vi "ImagenBinarizada.vi"(11 "Refnum in":T1) -> (3 "Refnum out":T1(plugin-control))   [LabVIEW 2021]
uses:
  <vilib>/vision/Image Controls.llb/IMAQ Image.ctl
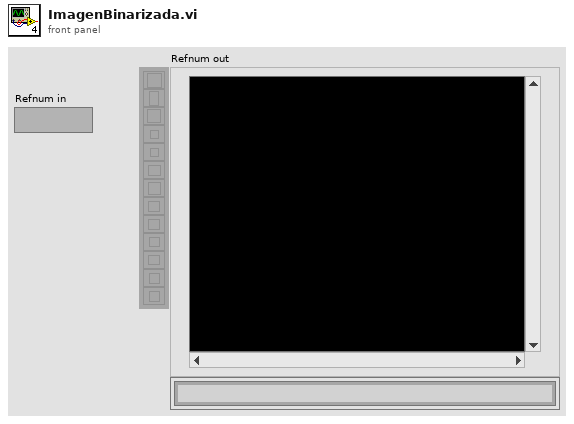
[diagram p1: front panel]
types:
  T1 = typedef "IMAQ Image.ctl" = refnum<image>
  T2 = typedef "Image Type" = u32
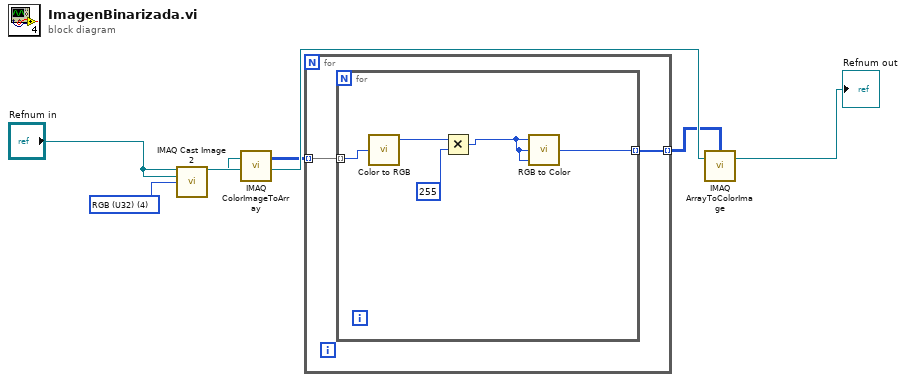
[diagram p0: block diagram]
diagram:
  w1 = T2 4 items=["Grayscale (U8)", "Grayscale (I16)", "Grayscale (SGL)", "Complex (CSG)", "RGB (U32)", "HSL (U32)", "RGB (U64)", "Grayscale (U16)"] ("Image Type")
  n1 = call "IMAQ Cast Image 2"("Image Src"="Refnum in", "Image Dst"="Refnum in", "Image Type"=w1) -> ("Image Dst Out"=w2:T1)  [unwired: 11 in, 1 out]
  n2 = call "IMAQ ColorImageToArray"("Image"=w2) -> ("Image Pixels (U32)"=w3:u32[][])  [unwired: 3 in, 2 out]
  n3 = for {
    tunnel: w3 -> [w8] mode=indexing
    tunnel: [w7] -> w4 mode=indexing
    n4 = for {
      tunnel: w8 -> [w13] mode=indexing
      tunnel: [w9] -> w7 mode=indexing
      n5 = call <vilib>:"Color to RGB.vi"("Color"=w13) -> ("Resolved Color"=w12:u32)  [unwired: 3 out]
      n6 = Multiply(x=w12, y=u32 255) -> (x*y=w10:u32)
      n7 = call <vilib>:"RGB to Color.vi"("B"=w10, "G"=w10, "R"=w10) -> ("Color"=w9:u32)
    }
  }
  n8 = call "IMAQ ArrayToColorImage"("Image Pixels (U32)"=w4, "Image"="Refnum in") -> ("Image Out"=→"Refnum out":T1)  [unwired: 3 in, 1 out]
